vi "RotateCoordinate.vi"(5 "Units":enum16{"mrad", "Radians", "Degrees"}(ring), 7 "Angle":dbl, 8 "y":dbl, 9 "x":dbl) -> (0 "y'":dbl, 1 "x'":dbl)   [LabVIEW 2016]
panel:
  out "cos(a)":dbl
  out "sin(a)":dbl
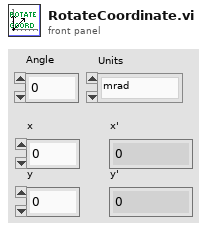
[diagram p1: front panel]
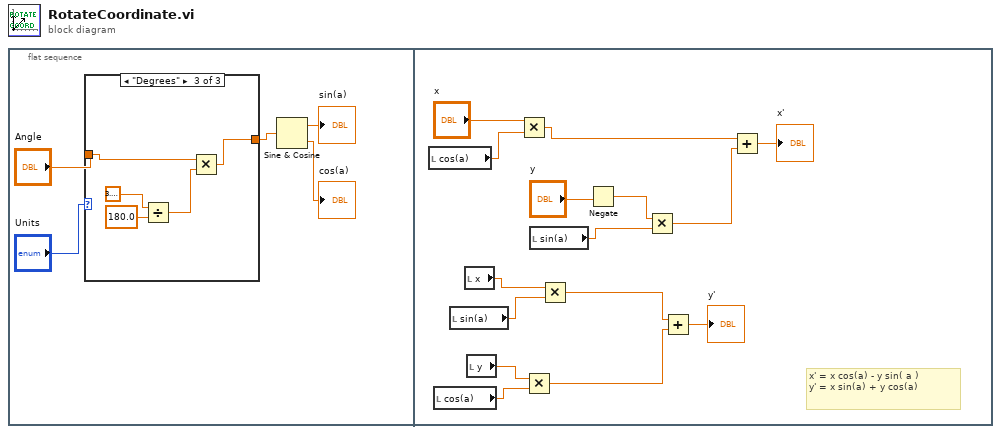
[diagram p0: block diagram]
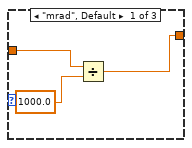
[diagram p2: hidden frame]
diagram:
  n1 = flat-sequence {
    frame #0 {
      n2 = case shown="\"Degrees\"" "Units" {
        tunnel: "Angle" -> [w8 w9 w11]
        tunnel: [w6 w9 w13] -> w2
        frame "mrad", Default {
          n3 = Divide(x=w8, y=1000.0) -> (x/y=w6:dbl)
        }
        frame "Radians" {
        }
        frame "Degrees" {
          n4 = Divide(x=3.141592653589793, y=180.0) -> (x/y=w12:dbl)
          n5 = Multiply(x=w11, y=w12) -> (x*y=w13:dbl)
        }
      }
      n6 = Sine & Cosine(0:w2) -> (1:→"sin(a)":dbl, 2:→"cos(a)":dbl)
    }
    frame #1 {
      # "x' = x cos(a) - y sin( a )\ny' = x sin(a) + y cos(a)"
      n7 = local read "cos(a)"() -> (w28:dbl)
      n8 = local read "cos(a)"() -> (w18:dbl)
      n9 = local read "sin(a)"() -> (w20:dbl)
      n10 = local read "x"() -> (w21:dbl)
      n11 = local read "y"() -> (w19:dbl)
      n12 = Multiply(x="x", y=w28) -> (x*y=w24:dbl)
      n13 = Multiply(x=w19, y=w18) -> (x*y=w16:dbl)
      n14 = local read "sin(a)"() -> (w26:dbl)
      n15 = Multiply(x=w21, y=w20) -> (x*y=w17:dbl)
      n16 = Negate(x="y") -> (-x=w25:dbl)
      n17 = Multiply(x=w25, y=w26) -> (x*y=w23:dbl)
      n18 = Add(x=w17, y=w16) -> (x+y=→"y'":dbl)
      n19 = Add(x=w24, y=w23) -> (x+y=→"x'":dbl)
    }
  }
